vi "Kroki Plot.vi"(8 "error in":errorcluster, 11 "Map":map{string, set{string}}(c390)) -> (0 "error out":errorcluster, 3 "Kroki Plot":picture)   [LabVIEW 2019, in "DependencyInspector.lvlib"]
uses:
  DependencyInspector.lvlib
  <vilib>/NI/Advanced HTTP Client/POST (Buffer).vi
  <vilib>/NI/Advanced HTTP Client/Session.lvclass
  <vilib>/wsapi/NI_WebServices.lvlib
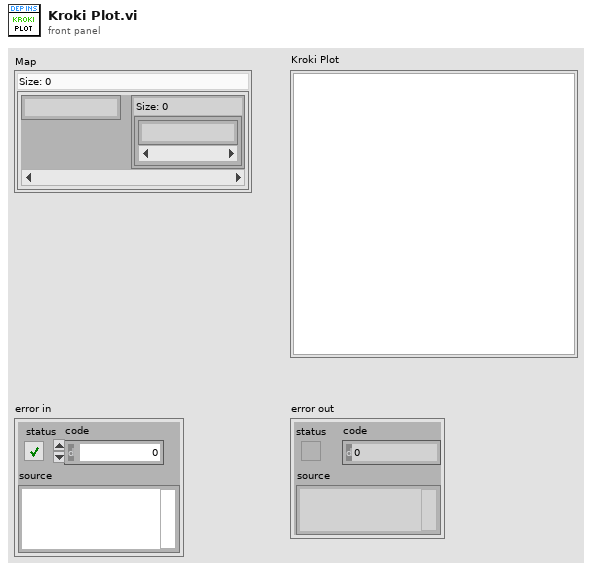
[diagram p1: front panel]
types:
  T1 = typedef "imagedata.ctl" = cluster{"image type":i32, "image depth":i32, "image":u8[], "mask":u8[], "colors":u32[], "Rectangle":cluster{"left":i16, "top":i16, "right":i16, "bottom":i16}}
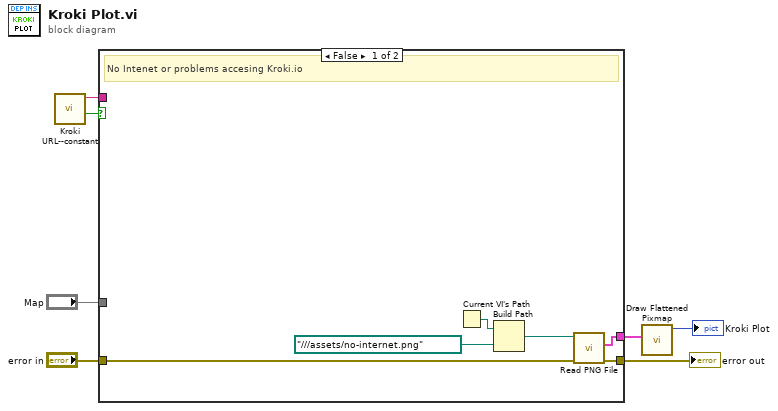
[diagram p0: block diagram]
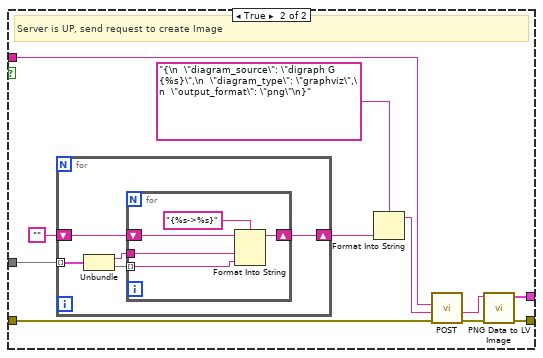
[diagram p2: hidden frame]
diagram:
  n1 = call "Kroki URL--constant.vi"() -> ("Server is UP"=w3:bool, "Kroki Full URL"=w5:string)  [unwired: 9 in, 1 out]
  n2 = case shown="False" w3 {
    tunnel: "error in" -> [w13 w23]
    tunnel: [w12 w22] -> w6
    tunnel: w5 -> [_ w20]
    tunnel: "Map" -> [_ w15]
    tunnel: [w8 w14] -> w2
    frame False {
      # "No Intenet or problems accesing Kroki.io"
      n3 = Current VI's Path() -> (path=w10:path)
      n4 = Build Path(base path=w10, name or relative path=path "../../../assets/no-internet.png") -> (appended path=w9:path)
      n5 = call <vilib>:"Read PNG File.vi"("error in (no error)"=w13, "path to PNG file"=w9) -> ("error out"=w12:errorcluster, "image data"=w8:T1)  [unwired: 7 in, 1 out]
    }
    frame True {
      # "Server is UP, send request to create Image"
      n6 = for {
        tunnel: w15 -> [w29] mode=indexing
        shift-right: [w26] -> w17
        shift-left: "" -> [w25]
        n7 = Unbundle(w29) -> (w27:string, w28:set{string})
        n8 = for {
          tunnel: w28 -> [w33] mode=indexing
          tunnel: w27 -> [w34]
          shift-right: [w31] -> w26
          shift-left: w25 -> [w30]
          n9 = Format Into String(format string="{%s->%s}", initial string=w30, w34, w33) -> (resulting string=w31:string)  [unwired: 1 in, 1 out]
        }
      }
      n10 = Format Into String(format string="{\n  \"diagram_source\": \"digraph G {%s}\",\n  \"diagram_type\": \"graphviz\",\n  \"output_format\": \"png\"\n}" ("buffer"), w17) -> (resulting string=w16:string)  [unwired: 2 in, 1 out]
      n11 = call-poly <vilib>:"POST.vi"("error in"=w23, "buffer"=w16, "url"=w20) -> ("error out"=w24:errorcluster, "body"=w21:string)  [unwired: 4 in, 3 out]
      n12 = call <vilib>:"PNG Data to LV Image.vi"("error in (no error)"=w24, "png data"=w21) -> ("error out"=w22:errorcluster, "image data"=w14:T1)  [unwired: 8 in]
    }
  }
  "error out" <- w6
  n13 = call <vilib>:"Draw Flattened Pixmap.vi"("image data"=w2) -> ("new picture"=→"Kroki Plot":picture)  [unwired: 8 in]
